vi "process_msg.vi"(11 "data":u8[](array[numeric])) -> (0 "valid":bool, 1 "size":u16, 2 "ID":u16, 3 "Addr":u16, 4 "data_out":u8[](array[numeric]))   [LabVIEW 2014]
uses:
  msg_state.ctl
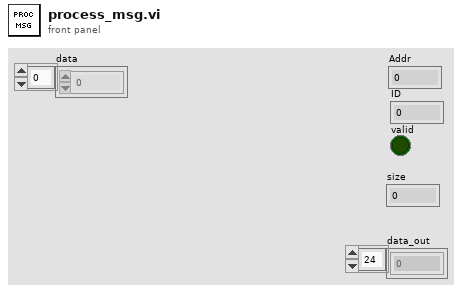
[diagram p1: front panel]
types:
  T1 = typedef "msg_state.ctl" = enum16{"Idle", "Sync1", "Sync2", "Addr", "ID", "Size", "Data", "CS", "Error"}
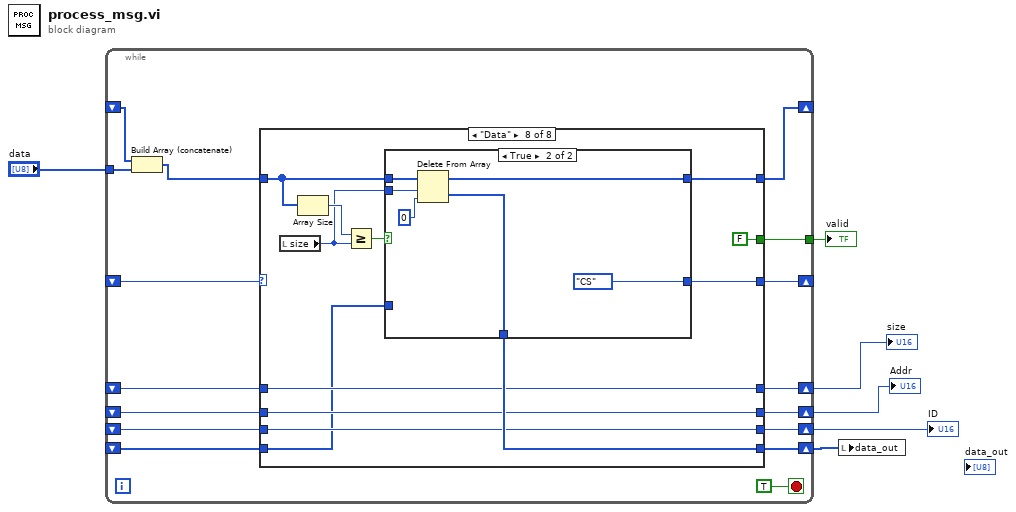
[diagram p0: block diagram]
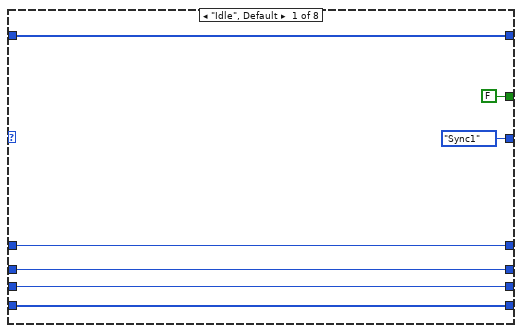
[diagram p2: hidden frame]
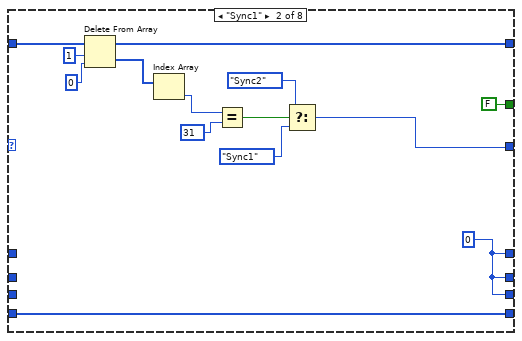
[diagram p3: hidden frame]
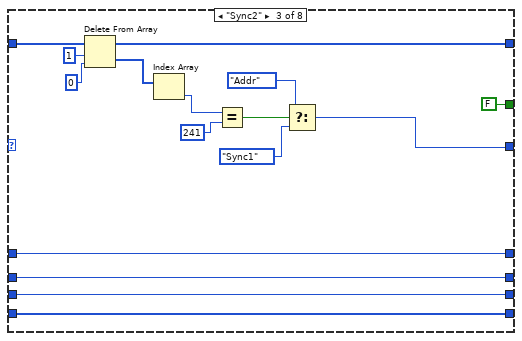
[diagram p4: hidden frame]
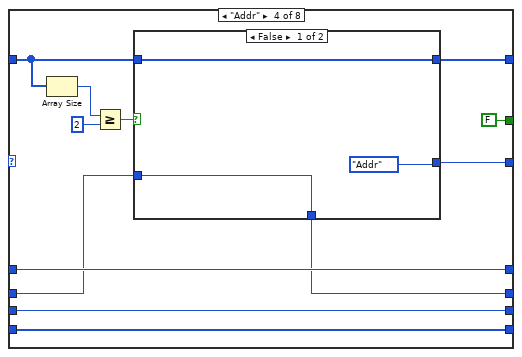
[diagram p5: hidden frame]
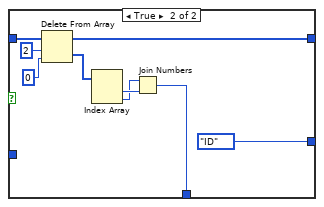
[diagram p6: hidden frame]
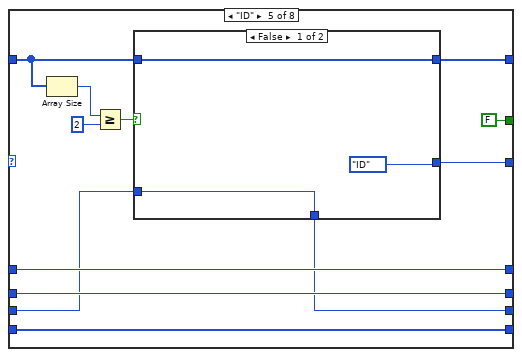
[diagram p7: hidden frame]
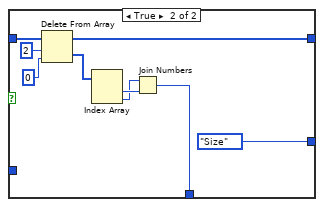
[diagram p8: hidden frame]
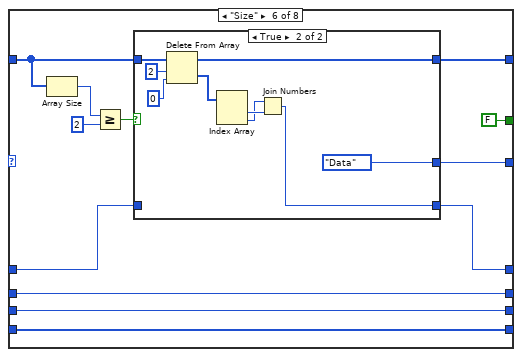
[diagram p9: hidden frame]
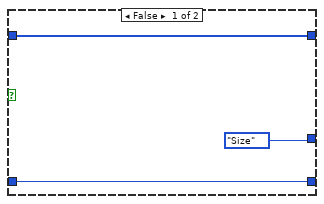
[diagram p10: hidden frame]
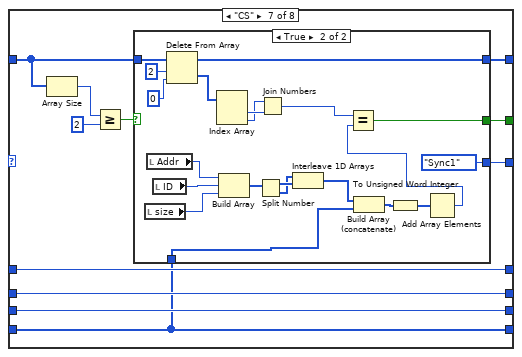
[diagram p11: hidden frame]
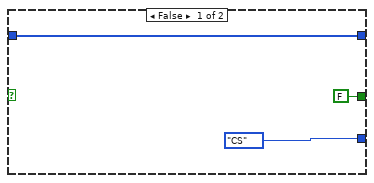
[diagram p12: hidden frame]
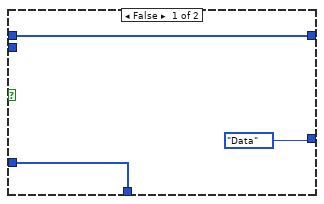
[diagram p13: hidden frame]
diagram:
  n1 = while {
    shift-right: [w20] -> _
    shift-left: _ -> [w19]
    shift-right: [w21] -> _
    shift-left: _ -> [w22]
    tunnel: "data" -> [w18]
    tunnel: [w16] -> w5
    shift-right: [w14] -> w1
    shift-left: _ -> [w13]
    shift-right: [w10] -> w3
    shift-left: _ -> [w9]
    shift-right: [w11] -> w2
    shift-left: _ -> [w7]
    shift-right: [w12] -> w4
    shift-left: _ -> [w8]
    stop <- TRUE stop-if-true
    n2 = Build Array (concatenate)(w19, w18) -> (w17:u8[])
    n3 = case shown="\"Data\"" w22 {
      tunnel: w17 -> [w27 w42 w58 w69 w93 w117 w140 w176]
      tunnel: [msg_state."Sync1" ("Enum") w34 w50 w71 w95 w119 w142 w178] -> w21
      tunnel: [w27 w33 w49 w70 w94 w118 w141 w177] -> w20
      tunnel: [FALSE FALSE FALSE FALSE FALSE FALSE w136 FALSE] -> w16
      tunnel: [w26 w30 w47 w64 w88 w112 w132 w171] -> w14
      tunnel: w13 -> [w26 w30 w47 w64 w88 w112 w132 w167]
      tunnel: [w24 w31 w45 w62 w86 w110 w134 w169] -> w12
      tunnel: [w23 w31 w44 w61 w85 w109 w133 w168] -> w11
      tunnel: [w25 w31 w46 w63 w87 w111 w135 w170] -> w10
      tunnel: w9 -> [w25 _ w46 w63 w87 w108 w135 w170]
      tunnel: w8 -> [w24 _ w45 w60 w86 w110 w134 w169]
      tunnel: w7 -> [w23 _ w44 w61 w84 w109 w133 w168]
      frame "Idle", Default {
      }
      frame "Sync1" {
        w31 = u16 0 ("Addr")
        n4 = Delete From Array(array=w42, length=1, index=0) -> (deleted portion=w40:u8[], array with subset deleted=w33:u8[])
        n5 = Index Array(array=w40) -> (element=w39:u8)  [unwired: 1 in]
        n6 = Equal?(x=w39, y=u8 31) -> (x = y?=w37:bool)
        n7 = Select(t=msg_state."Sync2" ("Enum"), s=w37, f=msg_state."Sync1" ("Enum")) -> (s? t:f=w34:T1)
      }
      frame "Sync2" {
        n8 = Delete From Array(array=w58, length=1, index=0) -> (deleted portion=w56:u8[], array with subset deleted=w49:u8[])
        n9 = Index Array(array=w56) -> (element=w55:u8)  [unwired: 1 in]
        n10 = Equal?(x=w55, y=u8 241) -> (x = y?=w53:bool)
        n11 = Select(t=msg_state."Addr" ("Enum"), s=w53, f=msg_state."Sync1" ("Enum")) -> (s? t:f=w50:T1)
      }
      frame "Addr" {
        n12 = Array Size(array=w69) -> (size(s)=w68:i32)
        n13 = Greater Or Equal?(x=w68, y=2) -> (x >= y?=w66:bool)
        n14 = case shown="False" w66 {
          tunnel: [msg_state."Addr" ("Enum") msg_state."ID" ("Enum")] -> w71
          tunnel: [w73 w80] -> w70
          tunnel: w69 -> [w73 w79]
          tunnel: [w72 w75] -> w62
          tunnel: w60 -> [w72 _]
          frame False {
          }
          frame True {
            n15 = Delete From Array(array=w79, length=2, index=0) -> (deleted portion=w81:u8[], array with subset deleted=w80:u8[])
            n16 = Index Array(array=w81) -> (element #1=w78:u8, element #2=w77:u8)  [unwired: 2 in]
            n17 = Join Numbers(hi=w77, lo=w78) -> ((hi.lo)=w75:u16)
          }
        }
      }
      frame "ID" {
        n18 = Array Size(array=w93) -> (size(s)=w92:i32)
        n19 = Greater Or Equal?(x=w92, y=2) -> (x >= y?=w90:bool)
        n20 = case shown="False" w90 {
          tunnel: [msg_state."ID" ("Enum") msg_state."Size" ("Enum")] -> w95
          tunnel: [w97 w104] -> w94
          tunnel: w93 -> [w97 w103]
          tunnel: [w96 w99] -> w85
          tunnel: w84 -> [w96 _]
          frame False {
          }
          frame True {
            n21 = Delete From Array(array=w103, length=2, index=0) -> (deleted portion=w105:u8[], array with subset deleted=w104:u8[])
            n22 = Index Array(array=w105) -> (element #1=w102:u8, element #2=w101:u8)  [unwired: 2 in]
            n23 = Join Numbers(hi=w101, lo=w102) -> ((hi.lo)=w99:u16)
          }
        }
      }
      frame "Size" {
        n24 = Array Size(array=w117) -> (size(s)=w116:i32)
        n25 = Greater Or Equal?(x=w116, y=2) -> (x >= y?=w114:bool)
        n26 = case shown="True" w114 {
          tunnel: [msg_state."Size" ("Enum") msg_state."Data" ("Enum")] -> w119
          tunnel: [w121 w128] -> w118
          tunnel: w117 -> [w121 w127]
          tunnel: [w120 w123] -> w111
          tunnel: w108 -> [w120 _]
          frame False {
          }
          frame True {
            n27 = Delete From Array(array=w127, length=2, index=0) -> (deleted portion=w129:u8[], array with subset deleted=w128:u8[])
            n28 = Index Array(array=w129) -> (element #1=w126:u8, element #2=w125:u8)  [unwired: 2 in]
            n29 = Join Numbers(hi=w125, lo=w126) -> ((hi.lo)=w123:u16)
          }
        }
      }
      frame "CS" {
        n30 = Array Size(array=w140) -> (size(s)=w139:i32)
        n31 = Greater Or Equal?(x=w139, y=2) -> (x >= y?=w137:bool)
        n32 = case shown="True" w137 {
          tunnel: [msg_state."CS" ("Enum") msg_state."Sync1" ("Enum")] -> w142
          tunnel: [w144 w163] -> w141
          tunnel: w140 -> [w144 w162]
          tunnel: [FALSE w147] -> w136
          tunnel: w132 -> [_ w146]
          frame False {
          }
          frame True {
            n33 = local read "size"() -> (w156:u16)
            n34 = local read "Addr"() -> (w158:u16)
            n35 = local read "ID"() -> (w157:u16)
            n36 = Delete From Array(array=w162, length=2, index=0) -> (deleted portion=w164:u8[], array with subset deleted=w163:u8[])
            n37 = Index Array(array=w164) -> (element #1=w161:u8, element #2=w160:u8)  [unwired: 2 in]
            n38 = Build Array(w158, w157, w156) -> (w155:u16[])
            n39 = Split Number(x=w155) -> (hi(x)=w154:u8[], lo(x)=w153:u8[])
            n40 = Join Numbers(hi=w160, lo=w161) -> ((hi.lo)=w149:u16)
            n41 = Interleave 1D Arrays(w153, w154) -> (w151:u8[])
            n42 = Build Array (concatenate)(w151, w146) -> (w150:u8[])
            n43 = To Unsigned Word Integer(number=w150) -> (unsigned 16bit integer=w152:u16[])
            n44 = Add Array Elements(numeric array=w152) -> (sum=w148:u16)
            n45 = Equal?(x=w149, y=w148) -> (x = y?=w147:bool)
          }
        }
      }
      frame "Data" {
        n46 = local read "size"() -> (w173:u16)
        n47 = Array Size(array=w176) -> (size(s)=w175:i32)
        n48 = Greater Or Equal?(x=w175, y=w173) -> (x >= y?=w174:bool)
        n49 = case shown="True" w174 {
          tunnel: [msg_state."Data" ("Enum") msg_state."CS" ("Enum")] -> w178
          tunnel: [w180 w186] -> w177
          tunnel: w176 -> [w180 w185]
          tunnel: w173 -> [_ w183]
          tunnel: [w179 w182] -> w171
          tunnel: w167 -> [w179 _]
          frame False {
          }
          frame True {
            n50 = Delete From Array(array=w185, length=w183, index=0) -> (deleted portion=w182:u8[], array with subset deleted=w186:u8[])
          }
        }
      }
    }
  }
  "Addr" <- w4
  "ID" <- w2
  "size" <- w3
  "valid" <- w5
  n51 = local write "data_out"(w1) -> ()
